vi "Salidas.vi"(11 "Class 2.lvclass":refnum<class "Class 2.lvclass">) -> (3 "Class 2.lvclass 2":refnum<class "Class 2.lvclass">)   [LabVIEW 2019, in "Class 2.lvclass"]
uses:
  Class 2.lvclass
  Class 2.lvclass/Class 2.ctl
  Datos Out.vi
  Datos In.vi
panel:
  out "MAQ DE ESTADOS":T1
  out "SALIDAS.SMAC DISTANCIA":dbl
  out "SALIDAS.SMAC g":dbl
  out "SALIDAS.MENSAJES":string
  out "SALIDAS.SAMAC AVANZANDO":bool
  out "SALIDAS.SEMAC RETORNANDO":bool
  out "SALIDAS.CILINDRO 2":bool
  out "SALIDAS.CILINDRO 1":bool
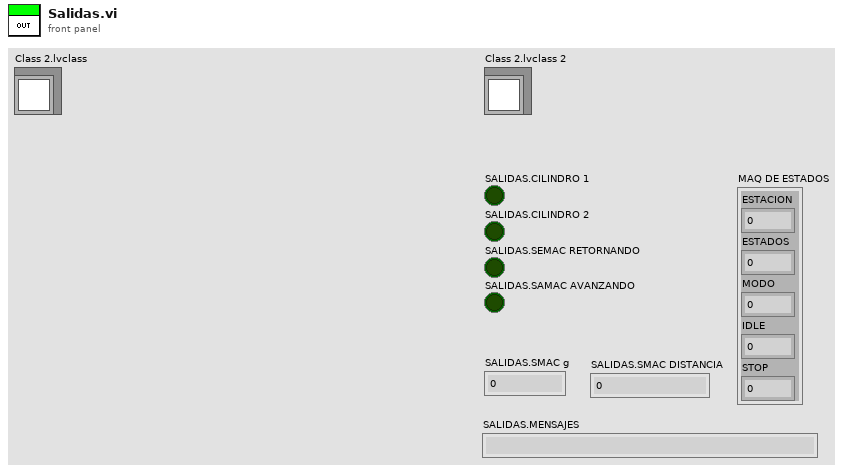
[diagram p1: front panel]
types:
  T1 = cluster{"ESTACION":i32, "ESTADOS":i16, "MODO":i16, "IDLE":i16, "STOP":i16}
  T2 = cluster{"SALIDAS.CILINDRO 1":bool, "SALIDAS.CILINDRO 2":bool, "SALIDAS.SEMAC RETORNANDO":bool, "SALIDAS.SAMAC AVANZANDO":bool, "Auto(off)/Manual(on)":bool, "HOME_CILINDRO_1":bool, "HOME_CILINDRO_2":bool, "AVANCE_CILINDRO_1":bool, "AVANCE_CILINDRO_2":bool, "PIEZA_EN_NIDO":bool, "BIMANUAL 2":bool, "BIMANUAL1":bool, "SIN CAMBIOS":bool, "CON  CAMBIOS":bool, "TESTER":bool, "MAQUINA EN ORIGEN":bool, "FALLA PRESENTE":bool}
  T3 = cluster{"Test":bool, "CILINDRO _1":bool, "CILINDRO _2":bool, "SMAC_RETORNANDO":bool, "SMAC_AVANZANDO":bool, "MANUAL":bool, "EST_1":bool, "EST_2":bool, "EST_3":bool, "MOVER A ORIGEN":bool, "RESET":bool, "PARO":bool, "INICIO":bool, "DATA_CONTROL":cluster{"ESTACION_1":cluster{"ACEPTADA":bool, "MAXIMO":dbl, "MINIMO":dbl, "LECTURA":dbl}, "ESTACION_2":cluster{"ACEPTADA":bool, "MAXIMO":dbl, "MINIMO":dbl, "LECTURA":dbl}, "ESTACION_3":cluster{"ACEPTADA":bool, "MAXIMO":dbl, "MINIMO":dbl, "LECTURA":dbl}}, "INGENIERIA O PROCESO":bool}
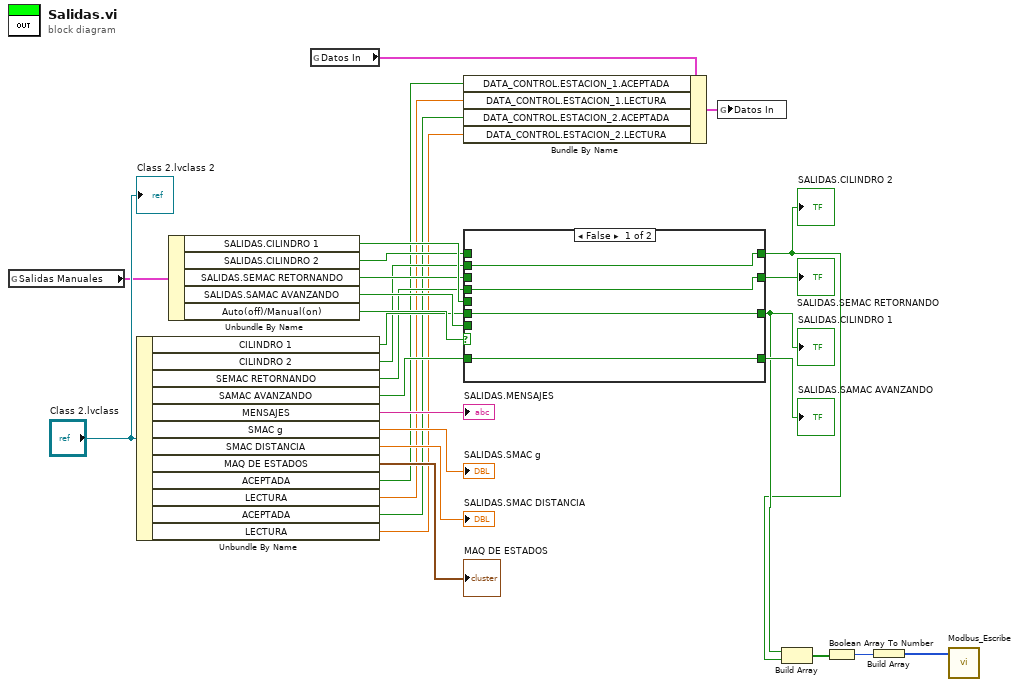
[diagram p0: block diagram]
diagram:
  n1 = global read "Datos Out.vi" "Salidas Manuales"() -> (w14:T2)
  n2 = Unbundle By Name("Class 2.lvclass") -> ("CILINDRO 1"=w19:bool, "CILINDRO 2"=w18:bool, "SEMAC RETORNANDO"=w17:bool, "SAMAC AVANZANDO"=w16:bool, "MENSAJES"=→"SALIDAS.MENSAJES":string, "SMAC g"=→"SALIDAS.SMAC g":dbl, "SMAC DISTANCIA"=→"SALIDAS.SMAC DISTANCIA":dbl, "MAQ DE ESTADOS"=→"MAQ DE ESTADOS":T1, "ACEPTADA"=w11:bool, "LECTURA"=w10:dbl, "ACEPTADA"=w9:bool, "LECTURA"=w8:dbl)
  n3 = Unbundle By Name(w14) -> ("SALIDAS.CILINDRO 1"=w23:bool, "SALIDAS.CILINDRO 2"=w22:bool, "SALIDAS.SEMAC RETORNANDO"=w21:bool, "SALIDAS.SAMAC AVANZANDO"=w20:bool, "Auto(off)/Manual(on)"=w24:bool)
  n4 = global read "Datos In.vi" "Datos In"() -> (w12:T3)
  n5 = Bundle By Name(cluster=w12, "DATA_CONTROL.ESTACION_1.ACEPTADA"=w11, "DATA_CONTROL.ESTACION_1.LECTURA"=w10, "DATA_CONTROL.ESTACION_2.ACEPTADA"=w9, "DATA_CONTROL.ESTACION_2.LECTURA"=w8) -> (w13:T3)
  n6 = case shown="False" w24 {
    tunnel: w23 -> [_ w36]
    tunnel: w22 -> [_ w35]
    tunnel: w21 -> [_ w34]
    tunnel: w20 -> [_ w33]
    tunnel: w19 -> [w32 _]
    tunnel: w18 -> [w31 _]
    tunnel: w17 -> [w30 _]
    tunnel: w16 -> [w29 _]
    tunnel: [w32 w36] -> w5
    tunnel: [w31 w35] -> w4
    tunnel: [w30 w34] -> w7
    tunnel: [w29 w33] -> w6
    frame False {
    }
    frame True {
    }
  }
  "SALIDAS.CILINDRO 1" <- w5
  "SALIDAS.CILINDRO 2" <- w4
  "SALIDAS.SEMAC RETORNANDO" <- w7
  "SALIDAS.SAMAC AVANZANDO" <- w6
  n7 = global write "Datos In.vi" "Datos In"(w13) -> ()
  n8 = Build Array(w5, w4) -> (w3:bool[])
  n9 = Boolean Array To Number(Boolean array=w3) -> (number=w2:u32)
  n10 = Build Array(w2) -> (w1:u32[])
  n11 = call "Modbus_Escribe.vi"("register values"=w1) -> ()  [unwired: 9 in]
  "Class 2.lvclass 2" <- "Class 2.lvclass"
